vi "Store.vi"(8 "error in (no error)":errorcluster, 11 "Persistent Path Selector in":refnum<class "MGI Persistent Path Selector.lvclass">) -> (0 "error out":errorcluster, 2 "String":string)   [LabVIEW 2016, in "MGI Persistent Path Selector.lvclass"]
doc: "Saves the persistent data of the class to a string.\n\nAuthored by Shawn Walpole\nsupport@mooregoodideas.com\nwww.mooregoodideas.com\n\nCopyright (c) 2013, Moore Good Ideas, Inc.\n\nAll rights reserved.\n\nRedistribution and use in source and binary forms, with or without modification, are permitted provided that the following conditions are met:\n\n * Redistributions of source code must retain the above copyright notice, this list of conditions and the following disclaimer.\n * Redistributions in binary form must reproduce the above copyright notice, this list of conditions and the following disclaimer in the documentation and/or other materials provided with the distribution.\n * Neither the name of Moore Good Ideas, Inc. nor the names of its contributors may be used to endorse or promote products derived from this software without specific prior written permission.\n\nTHIS SOFTWARE IS PROVIDED BY THE COPYRIGHT HOLDERS AND CONTRIBUTORS \"AS IS\" AND ANY EXPRESS OR IMPLIED WARRANTIES, INCLUDING, BUT NOT LIMITED TO, THE IMPLIED WARRANTIES OF MERCHANTABILITY AND FITNESS FOR A PARTICULAR PURPOSE ARE DISCLAIMED. IN NO EVENT SHALL THE COPYRIGHT OWNER OR CONTRIBUTORS BE LIABLE FOR ANY DIRECT, INDIRECT, INCIDENTAL, SPECIAL, EXEMPLARY, OR CONSEQUENTIAL DAMAGES (INCLUDING, BUT NOT LIMITED TO, PROCUREMENT OF SUBSTITUTE GOODS OR SERVICES; LOSS OF USE, DATA, OR PROFITS; OR BUSINESS INTERRUPTION) HOWEVER CAUSED AND ON ANY THEORY OF LIABILITY, WHETHER IN CONTRACT, STRICT LIABILITY, OR TORT (INCLUDING NEGLIGENCE OR OTHERWISE) ARISING IN ANY WAY OUT OF THE USE OF THIS SOFTWARE, EVEN IF ADVISED OF THE POSSIBILITY OF SUCH DAMAGE."
uses:
  <userlib>/_MGI/User Interface/Path Selector XControl/Class Hierarchy/Persistent Path Selector/MGI Persistent Path Selector.lvclass
  <userlib>/_MGI/User Interface/Path Selector XControl/Class Hierarchy/Persistent Path Selector/MGI Persistent Path Selector.lvclass/MGI Persistent Path Selector.ctl
  <userlib>/_MGI/User Interface/Path Selector XControl/Class Hierarchy/MGI Path Selector.lvclass
  <vilib>/Utility/VariantDataType/VariantType.lvlib
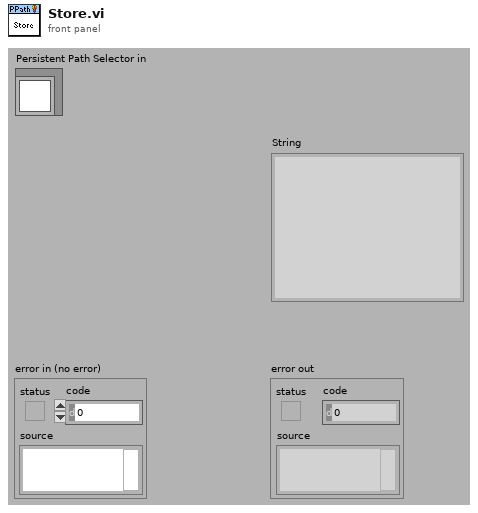
[diagram p1: front panel]
types:
  T1 = typedef "MGI Persistent Path Selector.lvclass/Persistent Data Cluster.ctl" = cluster{"Initial Path":path, "INI Path":path, "INI Section":string, "Select Option?":bool, "Explorer Option?":bool, "Recurse?":bool, "Allow New?":bool, "Filter":string}
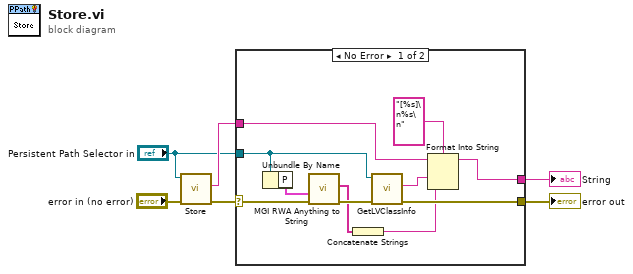
[diagram p0: block diagram]
diagram:
  n1 = call-parent "Store.vi"("error in (no error)"="error in (no error)", "Path Selector in"="Persistent Path Selector in") -> ("error out"=w4:errorcluster, "String"=w5:string)  [unwired: 8 in]
  n2 = case shown="No Error" w4 {
    selector: w4 -> [w13 w18]
    tunnel: [w17 w18] -> w2
    tunnel: "Persistent Path Selector in" -> [w16 _]
    tunnel: [w8 _] -> w1
    tunnel: w5 -> [w7 _]
    frame No Error {
      n3 = Unbundle By Name(w16) -> ("P"=w12:T1)
      n4 = call <userlib>:"MGI RWA Anything to String.vi"("Error In"=w13, "Anything"=w12) -> ("Error Out"=w11:errorcluster, "Strings[]"=w10:string[])  [unwired: 6 in, 2 out]
      n5 = Concatenate Strings(w10) -> (w9:string)
      n6 = call <vilib>:"GetLVClassInfo.vi"("error in (no error)"=w11, "Variant"=w16) -> ("error out"=w17:errorcluster, "LV Class File Name"=w14:string)  [unwired: 7 in, 1 out]
      n7 = Format Into String(format string="[%s]\n%s\n", initial string=w7, w14, w9) -> (resulting string=w8:string)  [unwired: 1 in, 1 out]
    }
    frame Error {
    }
  }
  "error out" <- w2
  "String" <- w1
